vi "Teleop.vi"(10 "Match Info":T1={"Autonomous Elapsed Seconds"=0.0, "TeleOp Elapsed Seconds"=0.0, "Disabled Elapsed Seconds"=0.0, "Visited Autonomous"=FALSE, "Visited TeleOp"=FALSE, "Visited Disabled"=FALSE, "Autonomous Settings"={"Autonomous Style"=enum."Independent", "VI Refnum"=refnum}}, 11 "Call Context":T2) -> ()   [LabVIEW 2012]
doc: "This VI is called for each TeleOp packet received from the DS where the robot is not disabled. It is often used to read from the joysticks and update I/O or to update setpoints for timed control loops. It should complete and return within 20 milliseconds or it may miss DS packets."
uses:
  <vilib>/Rock Robotics/WPI/DriverStation/WPI_DriverStationDerivedRobotMode.ctl
  <vilib>/Rock Robotics/WPI/DriverStation/WPI_DriverStationMatch Info.ctl
  <vilib>/Rock Robotics/WPI/Relay/WPI_RelayValue.ctl
  Robot Global Data.vi
  <vilib>/Rock Robotics/WPI/Joystick/WPI_JoystickGetSetRefNum.vi
  <vilib>/Rock Robotics/WPI/RobotDrive/WPI_RobotDriveGetSetRefNum.vi
panel:
  out "Percent of Motor Power":dbl(knob) scale=0.0..100.0
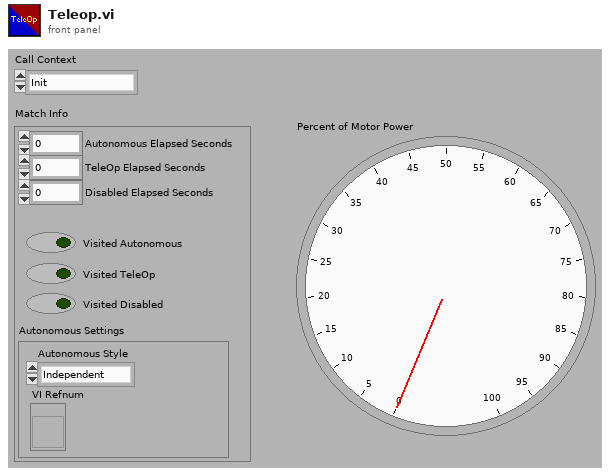
[diagram p1: front panel]
types:
  T1 = typedef "WPI_DriverStationMatch Info.ctl" = cluster{"Autonomous Elapsed Seconds":dbl, "TeleOp Elapsed Seconds":dbl, "Disabled Elapsed Seconds":dbl, "Visited Autonomous":bool, "Visited TeleOp":bool, "Visited Disabled":bool, "Autonomous Settings":cluster{"Autonomous Style":enum16{"Iterative", "Independent"}, "VI Refnum":refnum<vi>}}
  T2 = typedef "WPI_DriverStationDerivedRobotMode.ctl" = enum16{"Init", "Execute", "Stop"}
  T3 = typedef "WPI_JoystickDevRef.ctl" = cluster{"Device":T4}
  T4 = typedef "WPI_JoystickDeviceEnum.ctl" = enum16{"USB 1", "USB 2", "USB 3", "USB 4", "Kinect 1", "Kinect 2"}
  T5 = typedef "WPI_JoystickButtonState.ctl" = cluster{"Button 1":bool, "Button 2":bool, "Button 3":bool, "Button 4":bool, "Button 5":bool, "Button 6":bool, "Button 7":bool, "Button 8":bool, "Button 9":bool, "Button 10":bool, "Button 11":bool, "Button 12":bool}
  T6 = cluster{"axis 1 (x)":dbl, "axis 2 (y)":dbl, "axis 3 (throttle)":dbl, "axis 4":dbl, "axis 5":dbl, "axis 6":dbl}
  T7 = typedef "WPI_DigitalInputDevRef.ctl" = cluster{"DevStatus":errorcluster, "DIO Channel":T8, "Digital Module":T9}
  T8 = typedef "FPGA_DIOChannel.ctl" = enum8{"DIO 1", "DIO 2", "DIO 3", "DIO 4", "DIO 5", "DIO 6", "DIO 7", "DIO 8", "DIO 9", "DIO 10", "DIO 11", "DIO 12", "DIO 13", "DIO 14", "Invalid"}
  T9 = typedef "FPGA_TypedefDigitalModule.ctl" = enum16{"Digital Module 1", "Digital Module 2"}
  T10 = typedef "WPI_RelayDevRef.ctl" = cluster{"DevStatus":errorcluster, "Relay Channel":T11, "Digital Module":T9, "Relay Direction":T12}
  T11 = typedef "FPGA_DIORelayChannel.ctl" = enum8{"Relay 1", "Relay 2", "Relay 3", "Relay 4", "Relay 5", "Relay 6", "Relay 7", "Relay 8", "Invalid"}
  T12 = typedef "WPI_RelayDirection.ctl" = enum16{"Both directions", "Forward only", "Reverse only"}
  T13 = typedef "WPI_RelayValue.ctl" = enum16{"Off", "On", "Forward", "Reverse"}
  T14 = typedef "WPI_ServoDeviceRef.ctl" = cluster{"DeviceStatus":errorcluster, "Digital Module":T9, "PWM Channel":T15, "DeadBand":T16}
  T15 = typedef "FPGA_DIOPWMChannel.ctl" = enum8{"PWM 1", "PWM 2", "PWM 3", "PWM 4", "PWM 5", "PWM 6", "PWM 7", "PWM 8", "PWM 9", "PWM 10", "Invalid"}
  T16 = typedef "WPI_PWMDeadband.ctl" = cluster{"Name":string, "maxPositivePwm":i32, "minPositivePwm":i32, "centerPwm":i32, "maxNegativePwm":i32, "minNegativePwm":i32, "angularRange":u16}
  T17 = typedef "WPI_MotorControlDeviceRef.ctl" = cluster{"DeviceStatus":errorcluster, "Type":enum16{"PWM", "CAN"}, "PWM":cluster{"Digital Module":T9, "PWM Channel":T15, "DeadBand":T16}, "CAN":cluster{"Device Number":u8, "Control Mode":T18, "Semaphore":T19, "Max Vout":dbl}, "Invert":bool, "TransformRef":T20, "InvTransformRef":T20}
  T18 = typedef "WPI_CANJaguar_ControlMode.ctl" = enum8{"Percent VBus", "Current", "Speed", "Position", "Voltage"}
  T19 = typedef "Semaphore RefNum" = refnum<k1>
  T20 = typedef "WPI_PWMTransform_ConPane.ctl" = refnum<vi>
  T21 = typedef "WPI_RobotDriveDevRef.ctl" = cluster{"DevStatus":errorcluster, "Motors[]":T17[], "Square Inputs":bool, "Max Output":dbl, "Isochronous":bool}
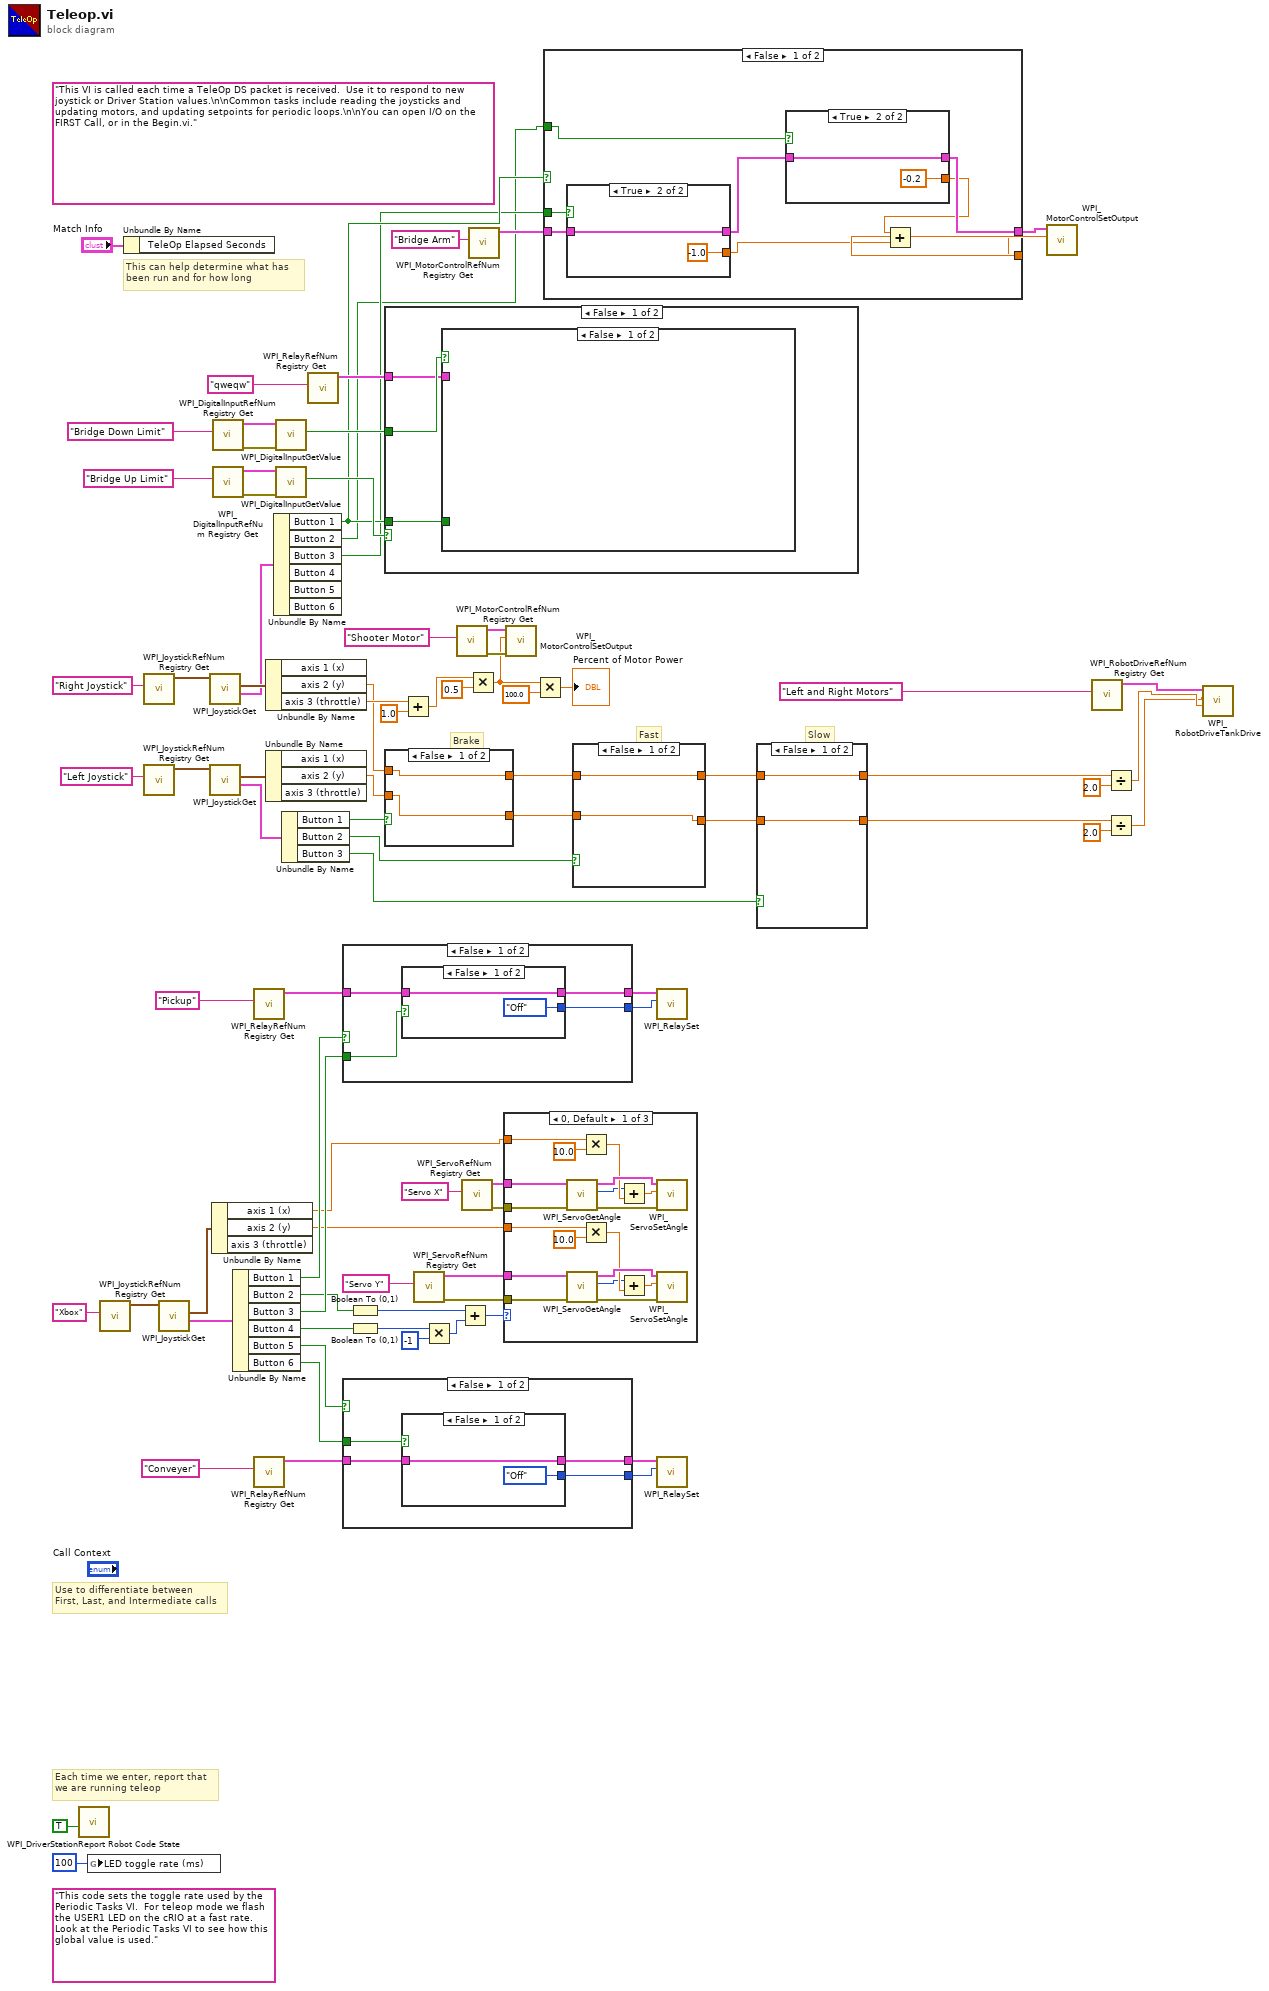
[diagram p0: block diagram]
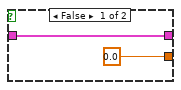
[diagram p2: hidden frame]
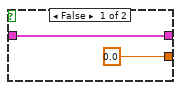
[diagram p3: hidden frame]
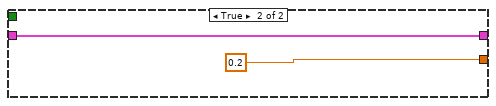
[diagram p4: hidden frame]
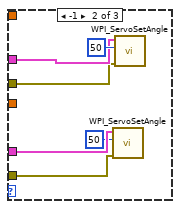
[diagram p5: hidden frame]
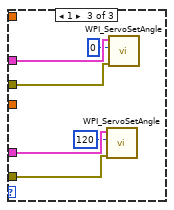
[diagram p6: hidden frame]
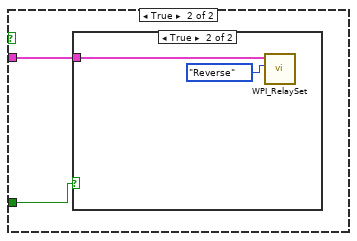
[diagram p7: hidden frame]
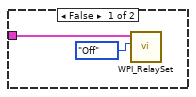
[diagram p8: hidden frame]
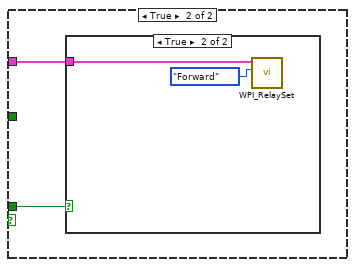
[diagram p9: hidden frame]
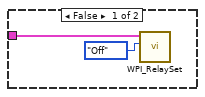
[diagram p10: hidden frame]
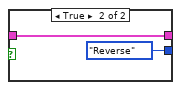
[diagram p11: hidden frame]
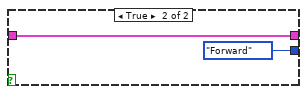
[diagram p12: hidden frame]
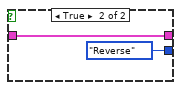
[diagram p13: hidden frame]
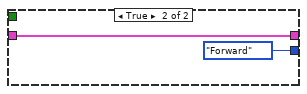
[diagram p14: hidden frame]
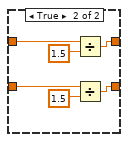
[diagram p15: hidden frame]
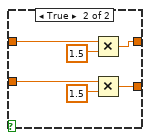
[diagram p16: hidden frame]
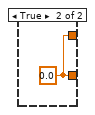
[diagram p17: hidden frame]
diagram:
  (unwired) "This code sets the toggle rate used by the Periodic Tasks VI.  For teleop mode we flash the USER1 LED on the cRIO at a fast rate.  Look at the Periodic Tasks VI to see how this global value is used."
  (unwired) "This VI is called each time a TeleOp DS packet is received.  Use it to respond to new joystick or Driver Station values.\n\nCommon tasks include reading the joysticks and updating motors, and updating setpoints for periodic loops.\n\nYou can open I/O on the FIRST Call, or in the Begin.vi."
  # "Slow"
  # "Fast"
  # "Brake"
  # "Each time we enter, report that\nwe are running teleop"
  # "Use to differentiate between\nFirst, Last, and Intermediate calls"
  # "This can help determine what has\nbeen run and for how long"
  n1 = call <vilib>:"WPI_DriverStationReport Robot Code State.vi"("TeleOp"=TRUE ("Autonomous")) -> ()  [unwired: 10 in, 1 out]
  n2 = global write "Robot Global Data.vi" "LED toggle rate (ms)"(u32 100 ("LED ms toggle rate")) -> ()
  n3 = call <vilib>:"WPI_JoystickRefNum Registry Get.vi"("refnum name"="Xbox") -> ("JoystickDevRef"=w56:T3)  [unwired: 1 in, 9 out]
  n4 = Unbundle By Name("Match Info") -> ()  [unwired: 1 out]
  n5 = call <vilib>:"WPI_JoystickRefNum Registry Get.vi"("refnum name"="Right Joystick") -> ("JoystickDevRef"=w66:T3)  [unwired: 1 in, 9 out]
  n6 = call <vilib>:"WPI_JoystickRefNum Registry Get.vi"("refnum name"="Left Joystick") -> ("JoystickDevRef"=w82:T3)  [unwired: 1 in, 9 out]
  n7 = call <vilib>:"WPI_JoystickGet.vi"("JoystickDevRef"=w56) -> ("Buttons"=w48:T5, "Axes"=w54:T6)  [unwired: 1 in, 4 out]
  n8 = call <vilib>:"WPI_JoystickGet.vi"("JoystickDevRef"=w66) -> ("Buttons"=w72:T5, "Axes"=w79:T6)  [unwired: 1 in, 4 out]
  n9 = call <vilib>:"WPI_JoystickGet.vi"("JoystickDevRef"=w82) -> ("Buttons"=w69:T5, "Axes"=w84:T6)  [unwired: 1 in, 4 out]
  n10 = Unbundle By Name(w54) -> ("axis 1 (x)"=w7:dbl, "axis 2 (y)"=w8:dbl)  [unwired: 1 out]
  n11 = call <vilib>:"WPI_DigitalInputRefNum Registry Get.vi"("refnum name"="Bridge Down Limit") -> ("error out"=w34:errorcluster, "DigitalInputDevRef"=w35:T7)  [unwired: 9 in]
  n12 = call <vilib>:"WPI_DigitalInputRefNum Registry Get.vi"("refnum name"="Bridge Up Limit") -> ("error out"=w32:errorcluster, "DigitalInputDevRef"=w33:T7)  [unwired: 9 in]
  n13 = Unbundle By Name(w48) -> ("Button 1"=w37:bool, "Button 2"=w25:bool, "Button 3"=w26:bool, "Button 4"=w24:bool, "Button 5"=w43:bool, "Button 6"=w42:bool)
  n14 = call <vilib>:"WPI_RelayRefNum Registry Get.vi"("refnum name"="Pickup") -> ("RelayDevRef"=w39:T10)  [unwired: 9 in, 1 out]
  n15 = call <vilib>:"WPI_RelayRefNum Registry Get.vi"("refnum name"="Conveyer") -> ("RelayDevRef"=w46:T10)  [unwired: 9 in, 1 out]
  n16 = Unbundle By Name(w79) -> ("axis 2 (y)"=w5:dbl, "axis 3 (throttle)"=w75:dbl)  [unwired: 1 out]
  n17 = Unbundle By Name(w84) -> ("axis 2 (y)"=w6:dbl)  [unwired: 2 out]
  n18 = Unbundle By Name(w72) -> ("Button 1"=w12:bool, "Button 2"=w1:bool, "Button 3"=w11:bool)  [unwired: 3 out]
  n19 = call <vilib>:"WPI_DigitalInputGetValue.vi"("error in (no error)"=w34, "DigitalInputDevRef"=w35) -> ("Value"=w29:bool)  [unwired: 7 in, 2 out]
  n20 = call <vilib>:"WPI_DigitalInputGetValue.vi"("error in (no error)"=w32, "DigitalInputDevRef"=w33) -> ("Value"=w31:bool)  [unwired: 7 in, 2 out]
  n21 = Unbundle By Name(w69) -> ("Button 1"=w68:bool, "Button 2"=w67:bool, "Button 3"=w63:bool)
  n22 = call <vilib>:"WPI_RelayRefNum Registry Get.vi"("refnum name"="qweqw") -> ("RelayDevRef"=w30:T10)  [unwired: 9 in, 1 out]
  n23 = case shown="False" w37 {
    tunnel: w39 -> [w89 w96]
    tunnel: [w88 w96] -> w41
    tunnel: [w90 WPI_RelayValue."Forward" ("RelayValue")] -> w40
    tunnel: w26 -> [w87 _]
    frame False {
      n24 = case shown="False" w87 {
        tunnel: [WPI_RelayValue."Off" ("RelayValue") WPI_RelayValue."Reverse" ("RelayValue")] -> w90
        tunnel: w89 -> [w92 w93]
        tunnel: [w92 w93] -> w88
        frame False {
        }
        frame True {
        }
      }
    }
    frame True {
    }
  }
  n25 = case shown="False" w43 {
    tunnel: w46 -> [w99 w106]
    tunnel: [w98 w106] -> w45
    tunnel: [w100 WPI_RelayValue."Forward" ("RelayValue")] -> w44
    tunnel: w42 -> [w97 _]
    frame False {
      n26 = case shown="False" w97 {
        tunnel: [WPI_RelayValue."Off" ("RelayValue") WPI_RelayValue."Reverse" ("RelayValue")] -> w100
        tunnel: w99 -> [w102 w103]
        tunnel: [w102 w103] -> w98
        frame False {
        }
        frame True {
        }
      }
    }
    frame True {
    }
  }
  n27 = Boolean To (0,1)(Boolean=w25) -> (0, 1=w19:i16)
  n28 = Boolean To (0,1)(Boolean=w24) -> (0, 1=w23:i16)
  n29 = case shown="False" w31 {
    tunnel: w12 -> [w108 w117]
    tunnel: w30 -> [w107 w116]
    tunnel: w29 -> [w109 _]
    frame False {
      n30 = case shown="False" w109 {
        tunnel: w107 -> [_ w111]
        tunnel: w108 -> [_ w110]
        frame False {
        }
        frame True {
          n31 = case shown="True" w110 {
            tunnel: w111 -> [w112 w114]
            frame False {
              n32 = call <vilib>:"WPI_RelaySet.vi"("RelayValue"=WPI_RelayValue."Off", "RelayDevRef"=w112) -> ()  [unwired: 8 in, 2 out]
            }
            frame True {
              n33 = call <vilib>:"WPI_RelaySet.vi"("RelayValue"=WPI_RelayValue."Reverse", "RelayDevRef"=w114) -> ()  [unwired: 8 in, 2 out]
            }
          }
        }
      }
    }
    frame True {
      n34 = case shown="True" w117 {
        tunnel: w116 -> [w118 w120]
        frame False {
          n35 = call <vilib>:"WPI_RelaySet.vi"("RelayValue"=WPI_RelayValue."Off", "RelayDevRef"=w118) -> ()  [unwired: 8 in, 2 out]
        }
        frame True {
          n36 = call <vilib>:"WPI_RelaySet.vi"("RelayValue"=WPI_RelayValue."Forward", "RelayDevRef"=w120) -> ()  [unwired: 8 in, 2 out]
        }
      }
    }
  }
  n37 = case shown="False" w68 {
    tunnel: [w123 w124] -> w71
    tunnel: [w122 w124] -> w70
    tunnel: w6 -> [w122 _]
    tunnel: w5 -> [w123 _]
    frame False {
    }
    frame True {
      w124 = 0.0 ("y")
    }
  }
  n38 = Add(x=w75, y=1.0) -> (x+y=w74:dbl)
  n39 = call <vilib>:"WPI_ServoRefNum Registry Get.vi"("refnum name"="Servo Y") -> ("error out"=w15:errorcluster, "ServoDeviceRef"=w16:T14)  [unwired: 9 in]
  n40 = Multiply(x=w23, y=i16 -1) -> (x*y=w20:i16)
  n41 = call <vilib>:"WPI_MotorControlRefNum Registry Get.vi"("refnum name"="Shooter Motor") -> ("error out"=w50:errorcluster, "MotorControlDevRef"=w51:T17)  [unwired: 9 in]
  n42 = Add(x=w19, y=w20) -> (x+y=w21:i16)
  n43 = call <vilib>:"WPI_ServoRefNum Registry Get.vi"("refnum name"="Servo X") -> ("error out"=w17:errorcluster, "ServoDeviceRef"=w18:T14)  [unwired: 9 in]
  n44 = Multiply(x=w74, y=0.5) -> (x*y=w49:dbl)
  n45 = call <vilib>:"WPI_MotorControlRefNum Registry Get.vi"("refnum name"="Bridge Arm") -> ("MotorControlDevRef"=w14:T17)  [unwired: 9 in, 1 out]
  n46 = case shown="0, Default" w21 {
    tunnel: w18 -> [w142 w147 w154]
    tunnel: w7 -> [w137 _ _]
    tunnel: w8 -> [w130 _ _]
    tunnel: w16 -> [w129 w145 w151]
    tunnel: w15 -> [w128 w144 w150]
    tunnel: w17 -> [w125 w146 w153]
    frame 0, Default {
      n47 = call <vilib>:"WPI_ServoGetAngle.vi"("ServoDeviceRef"=w142, "error in (no error)"=w125) -> ("ServoDeviceRef"=w141:T14, "Angle"=w138:u16, "error out"=w126:errorcluster)  [unwired: 6 in]
      n48 = call <vilib>:"WPI_ServoGetAngle.vi"("ServoDeviceRef"=w129, "error in (no error)"=w128) -> ("ServoDeviceRef"=w135:T14, "Angle"=w132:u16, "error out"=w127:errorcluster)  [unwired: 6 in]
      n49 = Multiply(x=w137, y=10.0) -> (x*y=w139:dbl)
      n50 = Multiply(x=w130, y=10.0) -> (x*y=w133:dbl)
      n51 = Add(x=w138, y=w139) -> (x+y=w136:dbl)
      n52 = Add(x=w132, y=w133) -> (x+y=w131:dbl)
      n53 = call <vilib>:"WPI_ServoSetAngle.vi"("error in (no error)"=w126, "Angle"=w136, "ServoDeviceRef"=w141) -> ()  [unwired: 7 in, 2 out]
      n54 = call <vilib>:"WPI_ServoSetAngle.vi"("error in (no error)"=w127, "Angle"=w131, "ServoDeviceRef"=w135) -> ()  [unwired: 7 in, 2 out]
    }
    frame -1 {
      n55 = call <vilib>:"WPI_ServoSetAngle.vi"("error in (no error)"=w144, "Angle"=50, "ServoDeviceRef"=w145) -> ()  [unwired: 7 in, 2 out]
      n56 = call <vilib>:"WPI_ServoSetAngle.vi"("error in (no error)"=w146, "Angle"=50, "ServoDeviceRef"=w147) -> ()  [unwired: 7 in, 2 out]
    }
    frame 1 {
      n57 = call <vilib>:"WPI_ServoSetAngle.vi"("error in (no error)"=w150, "Angle"=120, "ServoDeviceRef"=w151) -> ()  [unwired: 7 in, 2 out]
      n58 = call <vilib>:"WPI_ServoSetAngle.vi"("error in (no error)"=w153, "Angle"=0, "ServoDeviceRef"=w154) -> ()  [unwired: 7 in, 2 out]
    }
  }
  n59 = call <vilib>:"WPI_MotorControlSetOutput.vi"("error in (no error)"=w50, "Output"=w49, "MotorControlDevRef"=w51) -> ()  [unwired: 6 in, 3 out]
  n60 = Multiply(x=w49, y=100.0) -> (x*y=→"Percent of Motor Power":dbl)
  n61 = case shown="False" w12 {
    tunnel: w14 -> [w162 w172]
    tunnel: [w159 w172] -> w9
    tunnel: w11 -> [w161 _]
    tunnel: [w156 0.2 ("Output")] -> w10
    tunnel: w1 -> [w158 _]
    frame False {
      n62 = case shown="True" w161 {
        tunnel: w162 -> [w168 w170]
        tunnel: [w168 w170] -> w160
        tunnel: [0.0 ("Output") -1.0 ("Output")] -> w157
        frame False {
        }
        frame True {
        }
      }
      n63 = case shown="True" w158 {
        tunnel: w160 -> [w164 w166]
        tunnel: [w164 w166] -> w159
        tunnel: [0.0 ("Output") -0.2 ("Output")] -> w155
        frame False {
        }
        frame True {
        }
      }
      n64 = Add(x=w155, y=w157) -> (x+y=w156:dbl)
    }
    frame True {
    }
  }
  n65 = case shown="False" w67 {
    tunnel: w71 -> [w174 w179]
    tunnel: [w174 w180] -> w62
    tunnel: w70 -> [w173 w177]
    tunnel: [w173 w176] -> w60
    frame False {
    }
    frame True {
      n66 = Multiply(x=w179, y=1.5) -> (x*y=w180:dbl)
      n67 = Multiply(x=w177, y=1.5) -> (x*y=w176:dbl)
    }
  }
  n68 = call <vilib>:"WPI_RelaySet.vi"("RelayValue"=w40, "RelayDevRef"=w41) -> ()  [unwired: 8 in, 2 out]
  n69 = call <vilib>:"WPI_RelaySet.vi"("RelayValue"=w44, "RelayDevRef"=w45) -> ()  [unwired: 8 in, 2 out]
  n70 = case shown="False" w63 {
    tunnel: [w182 w187] -> w61
    tunnel: [w181 w188] -> w59
    tunnel: w62 -> [w182 w184]
    tunnel: w60 -> [w181 w183]
    frame False {
    }
    frame True {
      n71 = Divide(x=w184, y=1.5) -> (x/y=w187:dbl)
      n72 = Divide(x=w183, y=1.5) -> (x/y=w188:dbl)
    }
  }
  n73 = call <vilib>:"WPI_MotorControlSetOutput.vi"("Output"=w10, "MotorControlDevRef"=w9) -> ()  [unwired: 7 in, 3 out]
  n74 = call <vilib>:"WPI_RobotDriveRefNum Registry Get.vi"("refnum name"="Left and Right Motors") -> ("RobotDriveDevRef"=w4:T21)  [unwired: 1 in, 9 out]
  n75 = Divide(x=w61, y=2.0) -> (x/y=w3:dbl)
  n76 = Divide(x=w59, y=2.0) -> (x/y=w2:dbl)
  n77 = call <vilib>:"WPI_RobotDriveTankDrive.vi"("Right axis value"=w3, "Left axis value"=w2, "RobotDriveDevRef"=w4) -> ()  [unwired: 6 in, 3 out]
